vi "CopyImageARGBMaskARGB.vi"(8 "error in (no error)":errorcluster, 9 "ARGB Image Mask":refnum<data-value>, 10 "ARGB Image Destination":refnum<data-value>, 11 "ARGB Image Source":refnum<data-value>) -> (0 "error out":errorcluster, 3 "ARGB Image Destination (duplicate)":refnum<data-value>)   [LabVIEW 2020, in "g_ar_toolkit.image.lvlib"]
uses:
  g_ar_toolkit.image.lvlib
  3b1fb24f-4521-4d3d-a8b9-ed3d08148c99.vi
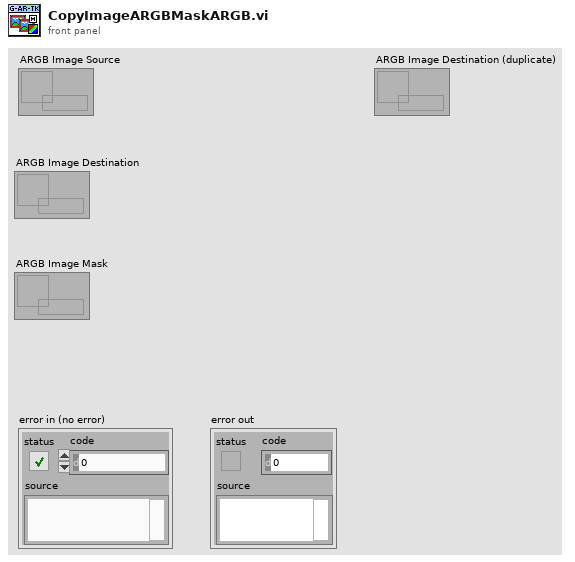
[diagram p1: front panel]
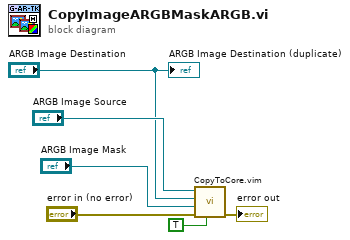
[diagram p0: block diagram]
diagram:
  n1 = call "CopyToCore.vim"("Has Mask"=TRUE, "error in (no error)"="error in (no error)", "Mask"="ARGB Image Mask", "Dst"="ARGB Image Destination", "Src"="ARGB Image Source") -> ("error out"=→"error out":errorcluster)  [unwired: 6 in]
  "ARGB Image Destination (duplicate)" <- "ARGB Image Destination"
